vi "Kc_correz_2024.vi"(0 "Temperature [K]":dbl=293.15 format="%.4g", 1 "Type of air":i32(listbox)=4, 2 "H2O molar fraction":dbl, 3 "CO2 content (ppm)":dbl=500.0) -> (4 "Cp0/R humid air":dbl=3.499501241139648, 5 "Gamma_simple corretto":dbl=1.4015054616866842 format="%.6g", 6 "Kc - correction Zuck wrong":dbl=5.7012386784904834e-05 format="%.7f", 7 "Kc - correction":dbl=-0.0010172235386579631 format="%.7f", 8 "Gamma_simple Zuckerwar (wrong)":dbl=1.4 format="%.6g", 9 "Gamma0 humid air":dbl=1.4000798173414988 format="%.6g")   [LabVIEW 2016]
uses:
  SOS_Global_2022.vi
panel:
  out "Kc - correction Zuck wrong / ppm":dbl=57.012386784904834 format="%#.0f"
  out "Kc - correction / ppm":dbl=-1017.2235386579631 format="%#.0f"
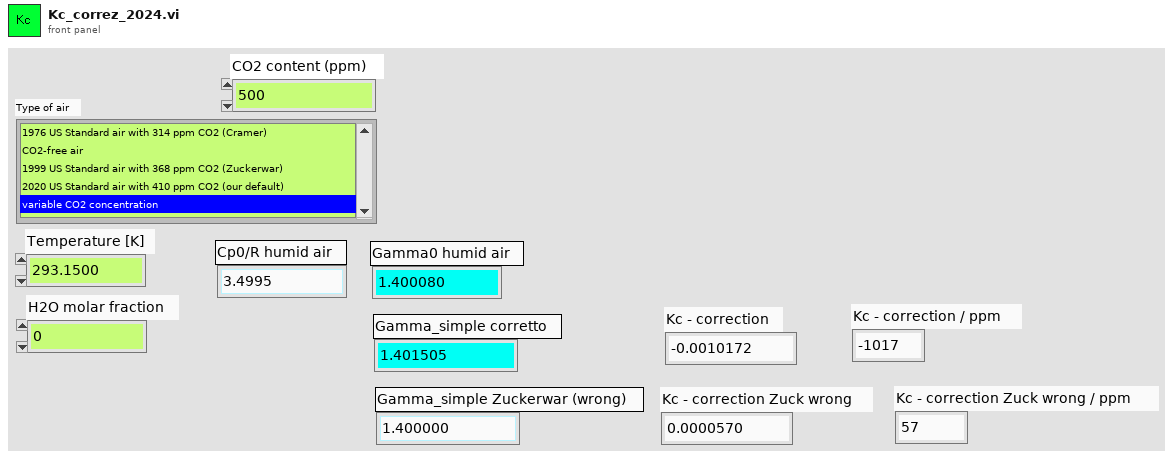
[diagram p1: front panel]
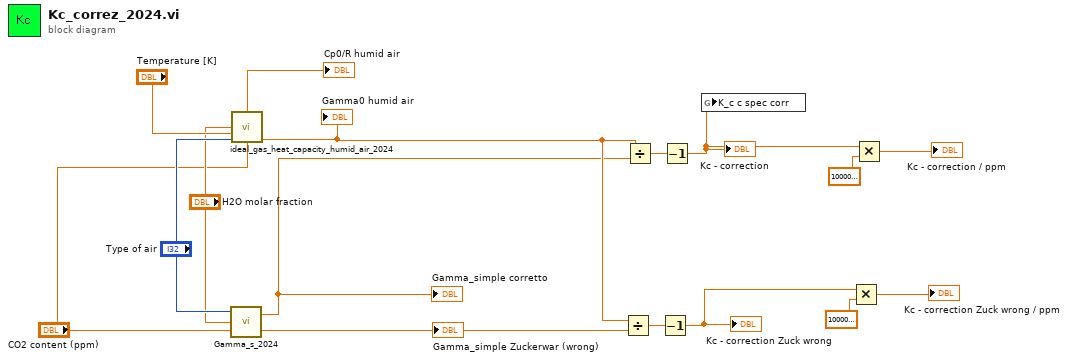
[diagram p0: block diagram]
diagram:
  n1 = call "Gamma_s_2024.vi"("CO2 content (ppm)"="CO2 content (ppm)", "xw molar fraction of water vapor"="H2O molar fraction", "Type of air"="Type of air") -> ("Gamma_s Zuckerwar (wrong)"=w16:dbl, "Gamma_s correct"=w5:dbl)
  "Gamma_simple Zuckerwar (wrong)" <- w16
  "Gamma_simple corretto" <- w5
  n2 = call "ideal_gas_heat_capacity_humid_air_2024.vi"("molar fraction of water vapor"="H2O molar fraction", "Temperature [K]"="Temperature [K]", "Type of air"="Type of air", "CO2 content (ppm)"="CO2 content (ppm)") -> ("Cp0/R humid air"=→"Cp0/R humid air":dbl, "Gamma0 humid air"=w6:dbl)  [unwired: 2 in, 8 out]
  "Gamma0 humid air" <- w6
  n3 = Divide(x=w6, y=w16) -> (x/y=w8:dbl)
  n4 = Divide(x=w6, y=w5) -> (x/y=w7:dbl)
  n5 = Decrement(x=w8) -> (x-1=w1:dbl)
  "Kc - correction Zuck wrong" <- w1
  n6 = Decrement(x=w7) -> (x-1=w4:dbl)
  "Kc - correction" <- w4
  n7 = global write "SOS_Global_2022.vi" "K_c c spec corr"(w4) -> ()
  n8 = Multiply(x=w1, y=1000000.0) -> (x*y=→"Kc - correction Zuck wrong / ppm":dbl)
  n9 = Multiply(x=w4, y=1000000.0) -> (x*y=→"Kc - correction / ppm":dbl)
